vi "Generate Grid Waypoints.vi"(5 "Camera Settings":T2, 7 "Altitude (m)":dbl, 9 "Overlap (%)":dbl, 11 "error in (no error)":errorcluster) -> (4 "Grid Waypoints":T1[](array[typedef]) {"Latitude" format="%#_10g"; "Longitude" format="%#_10g"}, 15 "error out":errorcluster)   [LabVIEW 2014]
uses:
  Settings File/Controls/Camera Settings.ctl
  Lat Long Conversion/Controls/PointLatLon.ctl
  Controls/Grid Waypoint States.ctl
  Reference/SubVI/Main Map Control Refernce.vi
  <vilib>/Analysis/geometry.llb/Point in Polygon (Scalar).vi
  <vilib>/Analysis/NI_AAL_Geometry.lvlib
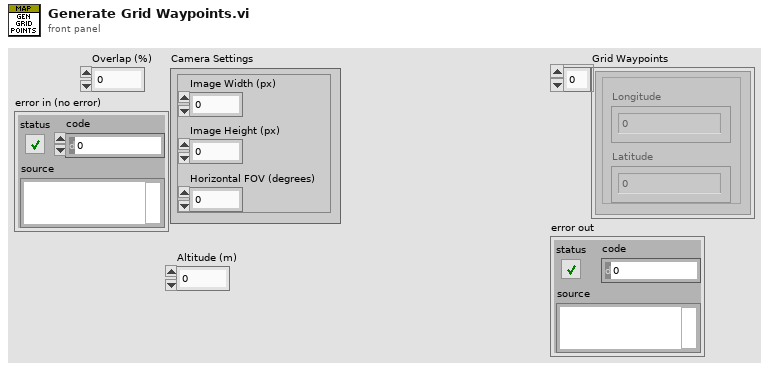
[diagram p1: front panel]
types:
  T1 = typedef "PointLatLon.ctl" = cluster{"Longitude":dbl, "Latitude":dbl}
  T2 = typedef "Camera Settings.ctl" = cluster{"Image Width (px)":dbl, "Image Height (px)":dbl, "Horizontal FOV (degrees)":dbl}
  T3 = typedef "Grid Waypoint States.ctl" = enum16{"Is Point in Polygon?", "Does Frame Intersect Polygon?", "Is Max LON Exceeded?", "Is Max/Min Lat Exceeded?", "Increment Lat", "Increment Lon", "Add Waypoint"}
  T4 = typedef "NI_AAL_Geometry.lvlib/Point in Polygon Position.ctl" = u16
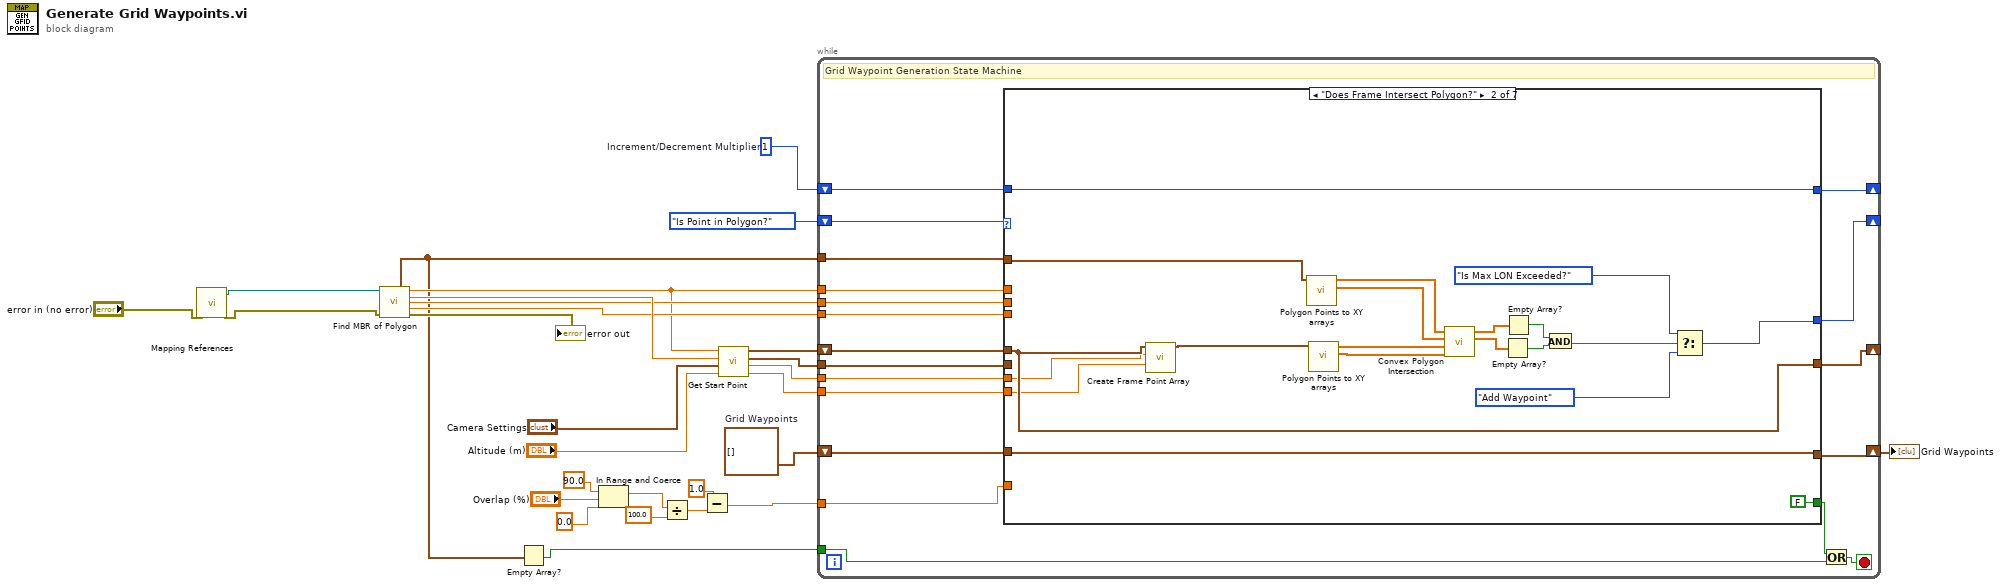
[diagram p0: block diagram]
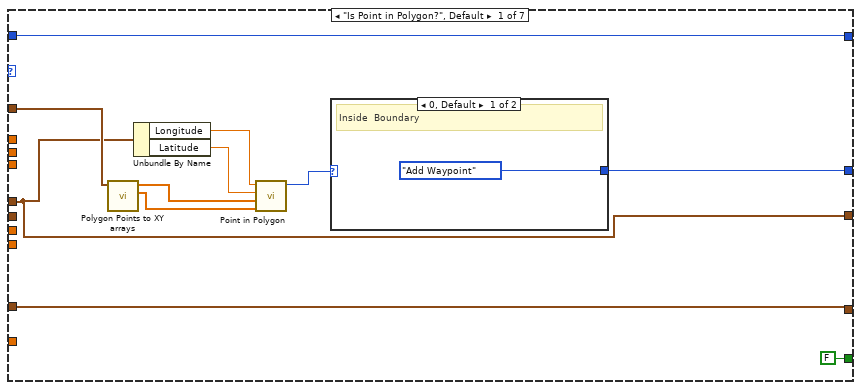
[diagram p2: hidden frame]
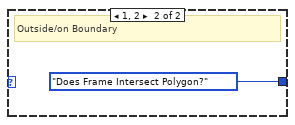
[diagram p3: hidden frame]
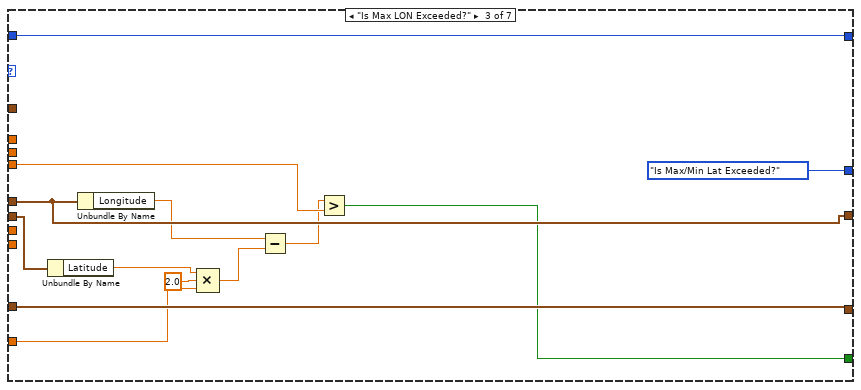
[diagram p4: hidden frame]
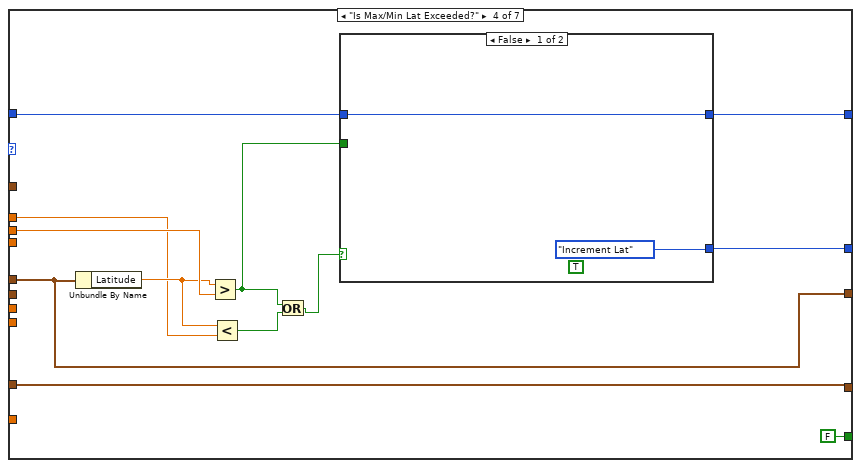
[diagram p5: hidden frame]
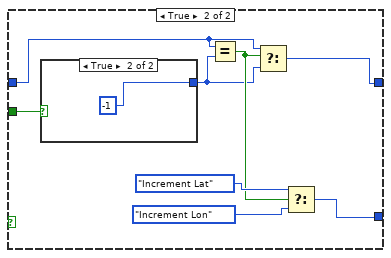
[diagram p6: hidden frame]
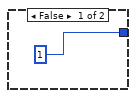
[diagram p7: hidden frame]
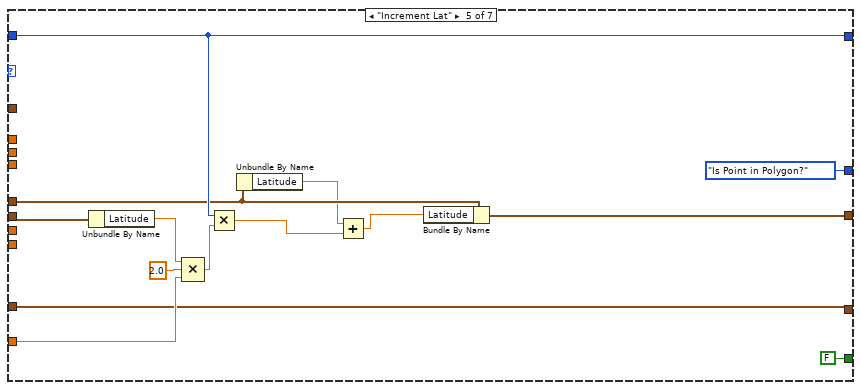
[diagram p8: hidden frame]
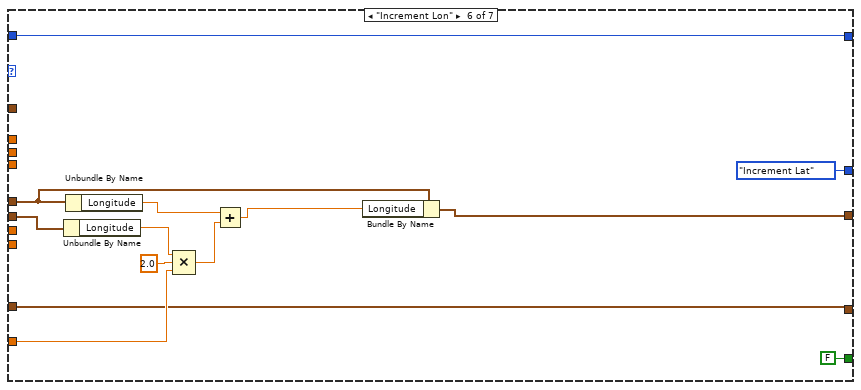
[diagram p9: hidden frame]
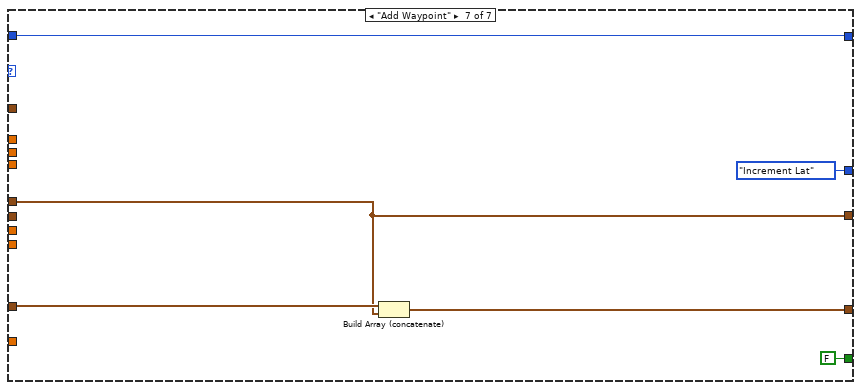
[diagram p10: hidden frame]
diagram:
  w16 = 1  # Increment/Decrement Multiplier
  w23 = T1[] []  # Grid Waypoints
  n1 = call-poly "Mapping References.vi"("Error In"="error in (no error)") -> ("Error Out"=w5:errorcluster, "Main Map Reference"=w4:refnum<k24>)  [unwired: 9 in]
  n2 = call "Find MBR of Polygon.vi"("Overlay Ref"=w4, "error in (no error)"=w5) -> ("Points of Polygon"=w2:T1[], "Min Lat"=w17:dbl, "Min Lon"=w28:dbl, "Max Lat"=w19:dbl, "Max Lon"=w18:dbl, "error out"=→"error out":errorcluster)  [unwired: 8 in]
  n3 = Empty Array?(array=w2) -> (empty?=w1:bool)
  n4 = In Range and Coerce(upper limit=90.0, x="Overlap (%)", lower limit=0.0) -> (coerced(x)=w12:dbl)  [unwired: 1 out]
  n5 = Divide(x=w12, y=100.0) -> (x/y=w9:dbl)
  n6 = Subtract(x=1.0, y=w9) -> (x-y=w8:dbl)
  n7 = call "Get Start Point.vi"("Altitude (m)"="Altitude (m)", "Camera Settings"="Camera Settings", "Lon"=w28, "Lat"=w17) -> ("Frame Height (m)"=w20:dbl, "Frame Width (m)"=w21:dbl, "Point Offset"=w22:T1, "Start Point"=w24:T1)  [unwired: 4 in]
  n8 = while {
    shift-right: [w42] -> _
    shift-left: Grid_Waypoint_States."Is Point in Polygon?" ("Grid Waypoint State") -> [w47]
    shift-right: [w35] -> _
    shift-left: w24 -> [w46]
    shift-right: [w32] -> w7
    shift-left: w23 -> [w44]
    tunnel: w22 -> [w45]
    tunnel: w2 -> [w43]
    tunnel: w21 -> [w41]
    tunnel: w20 -> [w40]
    tunnel: w19 -> [w39]
    tunnel: w18 -> [w38]
    tunnel: w17 -> [w37]
    shift-right: [w33] -> _
    shift-left: w16 -> [w36]
    tunnel: w8 -> [w34]
    tunnel: w1 -> [w29]
    stop <- w30 stop-if-true
    # "Grid Waypoint Generation State Machine"
    n9 = case shown="\"Does Frame Intersect Polygon?\"" w47 {
      tunnel: w46 -> [w55 w63 w93 w105 w129 w144 w145]
      tunnel: w45 -> [_ _ w85 _ w131 w143 _]
      tunnel: w44 -> [w49 w66 w90 w100 w119 w132 w149]
      tunnel: w43 -> [w58 w80 _ _ _ _ _]
      tunnel: [w51 w68 Grid_Waypoint_States."Is Max/Min Lat Exceeded?" ("Grid Waypoint State") w98 Grid_Waypoint_States."Is Point in Polygon?" ("f") Grid_Waypoint_States."Increment Lat" ("f") Grid_Waypoint_States."Increment Lat" ("f")] -> w42
      tunnel: w41 -> [_ w62 _ _ _ _ _]
      tunnel: w40 -> [_ w61 _ _ _ _ _]
      tunnel: w39 -> [_ _ _ w104 _ _ _]
      tunnel: w38 -> [_ _ w92 _ _ _ _]
      tunnel: w37 -> [_ _ _ w102 _ _ _]
      tunnel: [FALSE FALSE w86 FALSE FALSE FALSE FALSE] -> w31
      tunnel: w36 -> [w50 w67 w91 w94 w130 w133 w150]
      tunnel: [w55 w63 w93 w105 w125 w140 w145] -> w35
      tunnel: w34 -> [_ _ w82 _ w121 w136 _]
      tunnel: [w50 w67 w91 w101 w130 w133 w150] -> w33
      tunnel: [w49 w66 w90 w100 w119 w132 w148] -> w32
      frame "Is Point in Polygon?", Default {
        n10 = call "Polygon Points to XY arrays.vi"("Polygon Points"=w58) -> ("Y Array"=w57:dbl[], "X Array"=w56:dbl[])  [unwired: 9 in]
        n11 = Unbundle By Name(w55) -> ("Longitude"=w53:dbl, "Latitude"=w54:dbl)
        n12 = call-poly <vilib>:"Point in Polygon.vi"("Polygon Y"=w57, "Polygon X"=w56, "y"=w54, "x"=w53) -> ("position"=w52:T4)  [unwired: 6 in, 1 out]
        n13 = case shown="0, Default" w52 {
          tunnel: [Grid_Waypoint_States."Add Waypoint" ("Grid Waypoint State") Grid_Waypoint_States."Does Frame Intersect Polygon?" ("Grid Waypoint State")] -> w51
          frame 0, Default {
            # "Inside  Boundary"
          }
          frame 1, 2 {
            # "Outside/on Boundary"
          }
        }
      }
      frame "Does Frame Intersect Polygon?" {
        n14 = call "Create Frame Point Array.vi"("Height (m)"=w61, "Width (m)"=w62, "Origin Point"=w63) -> ("Frame Points"=w64:T1[])  [unwired: 8 in]
        n15 = call "Polygon Points to XY arrays.vi"("Polygon Points"=w80) -> ("Y Array"=w78:dbl[], "X Array"=w79:dbl[])  [unwired: 9 in]
        n16 = call "Polygon Points to XY arrays.vi"("Polygon Points"=w64) -> ("Y Array"=w76:dbl[], "X Array"=w77:dbl[])  [unwired: 9 in]
        n17 = call <vilib>:"Convex Polygon Intersection.vi"("Y 2"=w76, "X 2"=w77, "Y 1"=w78, "X 1"=w79) -> ("Intersection Y"=w74:dbl[], "Intersection X"=w75:dbl[])  [unwired: 5 in, 1 out]
        n18 = Empty Array?(array=w74) -> (empty?=w72:bool)
        n19 = Empty Array?(array=w75) -> (empty?=w73:bool)
        n20 = And(x=w73, y=w72) -> (x .and. y?=w71:bool)
        n21 = Select(t=Grid_Waypoint_States."Is Max LON Exceeded?", s=w71, f=Grid_Waypoint_States."Add Waypoint" ("Grid Waypoint State")) -> (s? t:f=w68:T3)
      }
      frame "Is Max LON Exceeded?" {
        n22 = Unbundle By Name(w85) -> ("Latitude"=w83:dbl)
        n23 = Unbundle By Name(w93) -> ("Longitude"=w88:dbl)
        n24 = Compound Arithmetic op=MULTIPLY(w83, 2.0 ("y"), w82) -> (w81:dbl)
        n25 = Subtract(x=w88, y=w81) -> (x-y=w87:dbl)
        n26 = Greater?(x=w87, y=w92) -> (0:w86:bool)
      }
      frame "Is Max/Min Lat Exceeded?" {
        n27 = Unbundle By Name(w105) -> ("Latitude"=w103:dbl)
        n28 = Greater?(x=w103, y=w104) -> (0:w96:bool)
        n29 = Less?(x=w103, y=w102) -> (x < y?=w99:bool)
        n30 = Or(x=w96, y=w99) -> (x .or. y?=w97:bool)
        n31 = case shown="False" w97 {
          tunnel: w94 -> [w107 w108]
          tunnel: [w107 w110] -> w101
          tunnel: w96 -> [_ w114]
          tunnel: [Grid_Waypoint_States."Increment Lat" ("f") w109] -> w98
          frame False {
            (unwired) TRUE
          }
          frame True {
            n32 = case shown="True" w114 {
              tunnel: [1 -1] -> w111
              frame False {
              }
              frame True {
              }
            }
            n33 = Equal?(x=w108, y=w111) -> (x = y?=w113:bool)
            n34 = Select(t=w108, s=w113, f=w111) -> (s? t:f=w110:i32)
            n35 = Select(t=Grid_Waypoint_States."Increment Lat" ("Grid Waypoint State"), s=w113, f=Grid_Waypoint_States."Increment Lon" ("Grid Waypoint State")) -> (s? t:f=w109:T3)
          }
        }
      }
      frame "Increment Lat" {
        n36 = Unbundle By Name(w131) -> ("Latitude"=w122:dbl)
        n37 = Compound Arithmetic op=MULTIPLY(w122, 2.0 ("y"), w121) -> (w120:dbl)
        n38 = Multiply(x=w130, y=w120) -> (x*y=w127:dbl)
        n39 = Unbundle By Name(w129) -> ("Latitude"=w128:dbl)
        n40 = Add(x=w128, y=w127) -> (x+y=w126:dbl)
        n41 = Bundle By Name(cluster=w129, "Latitude"=w126) -> (w125:T1)
      }
      frame "Increment Lon" {
        n42 = Unbundle By Name(w143) -> ("Longitude"=w139:dbl)
        n43 = Unbundle By Name(w144) -> ("Longitude"=w142:dbl)
        n44 = Compound Arithmetic op=MULTIPLY(w139, 2.0 ("y"), w136) -> (w137:dbl)
        n45 = Add(x=w142, y=w137) -> (x+y=w141:dbl)
        n46 = Bundle By Name(cluster=w144, "Longitude"=w141) -> (w140:T1)
      }
      frame "Add Waypoint" {
        n47 = Build Array (concatenate)(w149, w145) -> (w148:T1[])
      }
    }
    n48 = Or(x=w31, y=w29) -> (x .or. y?=w30:bool)
  }
  "Grid Waypoints" <- w7
